vi "getLockStatus.vi"(8 "error in":errorcluster, 11 "connection ID in":refnum<k5>) -> (0 "error out":errorcluster, 1 "locked":bool=TRUE, 2 "authorized":bool=TRUE, 3 "connection ID out":refnum<k5>)   [LabVIEW 2019]
panel:
  in  "Get Command":string="getLockStatus"
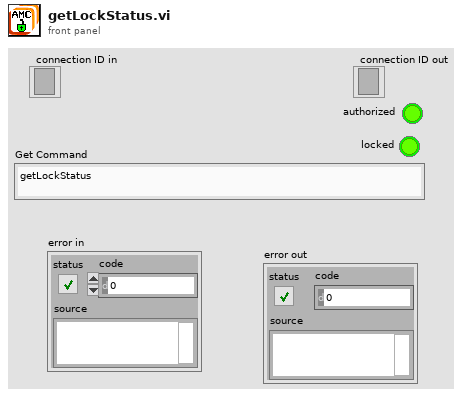
[diagram p1: front panel]
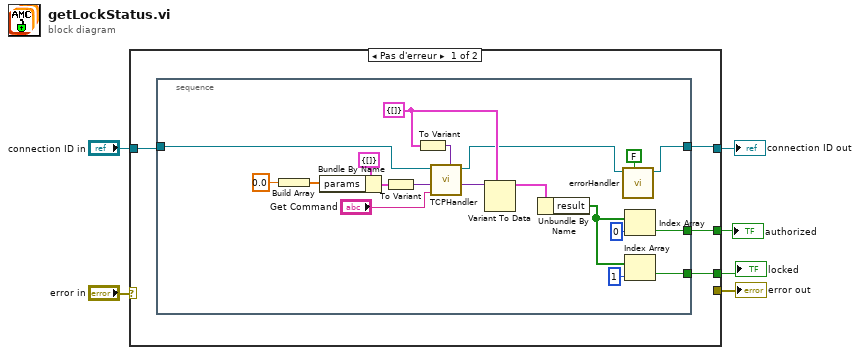
[diagram p0: block diagram]
diagram:
  n1 = case shown="Pas d'erreur" "error in" {
    selector: "error in" -> [_ w31]
    tunnel: [_ w31] -> w6
    tunnel: [w7 w30] -> w5
    tunnel: "connection ID in" -> [w8 w30]
    tunnel: [w10 _] -> w2
    tunnel: [w9 _] -> w1
    frame No Error {
      n2 = stacked-sequence {
        tunnel: [w11] -> w7
        tunnel: w8 -> [w22]
        tunnel: [w14] -> w9
        tunnel: [w13] -> w10
        frame #0 {
          w20 = cluster{"result":bool[]} {"result"=[]} ("input cluster")
          n3 = Build Array(0.0 ("element")) -> (w26:dbl[])
          n4 = Bundle By Name(cluster=cluster{"params":i16[]} {"params"=[]} ("input cluster"), "params"=w26) -> (w27:cluster{"params":i16[]})
          n5 = To Variant(anything=w27) -> (Variant=w28:variant)
          n6 = To Variant(anything=w20) -> (Variant=w21:variant)
          n7 = call "TCPHandler.vi"("result Types"=w21, "method"="Get Command", "params"=w28, "connection ID"=w22) -> ("result"=w24:variant, "connection ID"=w12:refnum<k5>)  [unwired: 5 in, 1 out]
          n8 = Variant To Data(type=w20, Variant=w24) -> (data=w29:cluster{"result":bool[]})  [unwired: 1 in, 1 out]
          n9 = Unbundle By Name(w29) -> ("result"=w15:bool[])
          n10 = call "errorHandler.vi"("show popup"=FALSE, "connection ID"=w12) -> ("connection ID"=w11:refnum<k5>)  [unwired: 8 in, 1 out]
          n11 = Index Array(array=w15, index=0) -> (element=w14:bool)
          n12 = Index Array(array=w15, index=1) -> (element=w13:bool)
        }
      }
    }
    frame Error {
    }
  }
  "error out" <- w6
  "locked" <- w2
  "connection ID out" <- w5
  "authorized" <- w1
